vi "histeresis.vi"() -> ()   [LabVIEW 2020]
panel:
  in  "x":dbl
  out "Valores":dbl
  in  "MAX":dbl
  in  "MIN":dbl
  out "Histeresis":bool
  out "Si está":bool
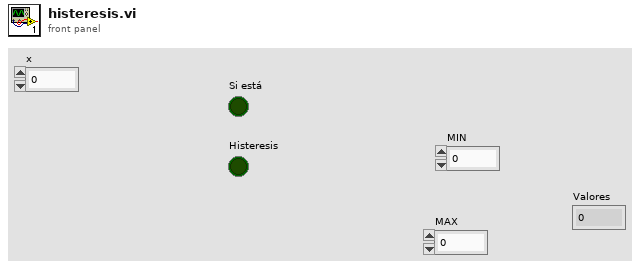
[diagram p1: front panel]
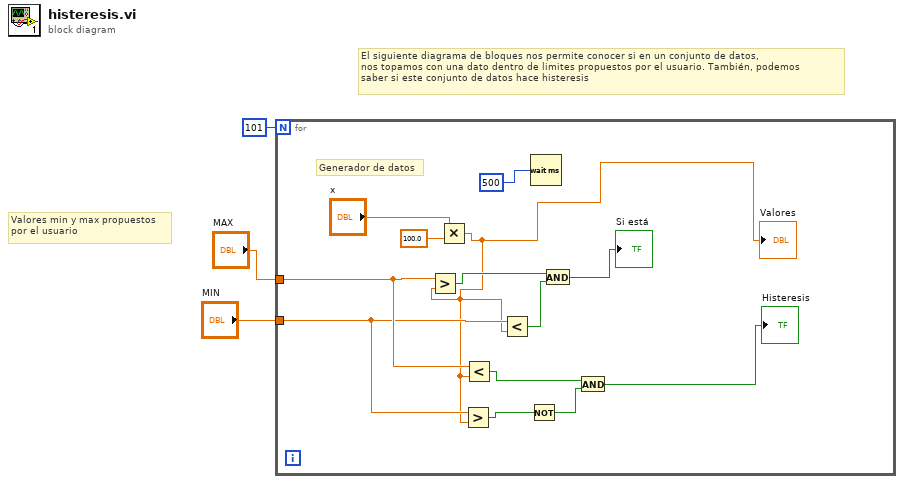
[diagram p0: block diagram]
diagram:
  # "Valores min y max propuestos\npor el usuario"
  # "El siguiente diagrama de bloques nos permite conocer si en un conjunto de datos, \nnos topamos con una dato dentro de limites propuestos por el usuario. También, podemos \nsaber si este conjunto de datos hace histeresis"
  n1 = for {
    N: 101 -> [_]
    tunnel: "MAX" -> [w11]
    tunnel: "MIN" -> [w10]
    # "Generador de datos"
    n2 = Multiply(x="x", y=100.0) -> (x*y=w9:dbl)
    "Valores" <- w9
    n3 = Greater?(x=w11, y=w9) -> (0:w13:bool)
    n4 = Greater?(x=w10, y=w9) -> (0:w7:bool)
    n5 = Less?(x=w11, y=w9) -> (x < y?=w8:bool)
    n6 = Less?(x=w10, y=w9) -> (x < y?=w12:bool)
    n7 = Not(x=w7) -> (.not. x?=w6:bool)
    n8 = Wait (ms)(milliseconds to wait=u32 500) -> ()  [unwired: 1 out]
    n9 = And(x=w13, y=w12) -> (x .and. y?=→"Si está":bool)
    n10 = And(x=w8, y=w6) -> (x .and. y?=→"Histeresis":bool)
  }
